vi "ULx Create Channel (DO-Digital Output).vi"(0 "task in":refnum<k24>, 5 "lines":refnum<k21>, 9 "line grouping":i32(ring)=1 items=["OneChannelForEachLine", "OneChannelForAllLines"], 11 "error in":errorcluster) -> (4 "task out":refnum<k24>, 15 "error out":errorcluster)   [LabVIEW 2020]
doc: "Creates channel(s) to generate digital signals. You can group digital lines into one digital channel or separate them into multiple digital channels. If you specify one or more entire ports in <B>lines</B> input by using port physical channel names, you cannot separate the ports into multiple channels. To separate ports into multiple channels, use this VI multiple times with a different port each time."
uses:
  C:/Users/William/Documents/LV 2020 builds/LeaktestDAQ/Source-v33/ULx_LV.dll
  ULx_LV.dll
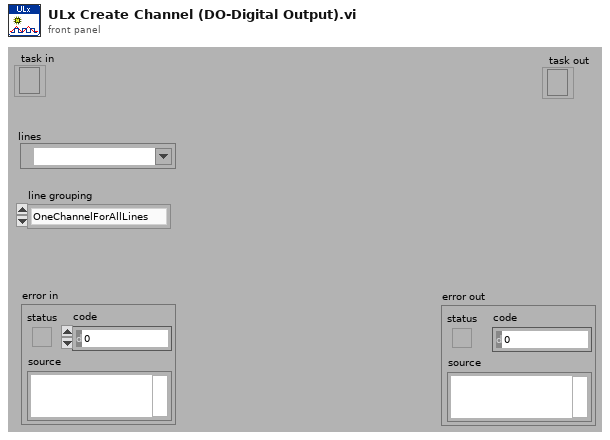
[diagram p1: front panel]
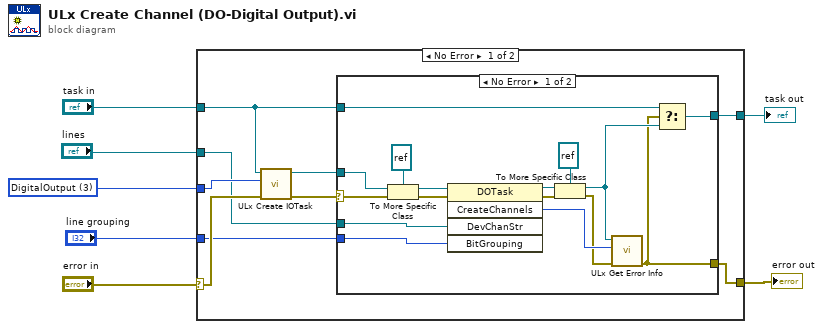
[diagram p0: block diagram]
diagram:
  w2 = 3 items=["AnalogInput", "AnalogOutput", "DigitalInput", "DigitalOutput", "CounterInput", "CounterOutput", "CompositeInput", "CompositeOutput", "TemperatureInput"] ("taskType")
  n1 = case shown="No Error" "error in" {
    selector: "error in" -> [w16 w36]
    tunnel: "task in" -> [w8 w35]
    tunnel: "lines" -> [w10 _]
    tunnel: w2 -> [w11 _]
    tunnel: [w14 w35] -> w5
    tunnel: [w13 w36] -> w4
    tunnel: "line grouping" -> [w9 _]
    frame No Error {
      n2 = call "ULx Create IOTask.vi"("error in"=w16, "taskType"=w11, "i/o task in"=w8) -> ("error out"=w15:errorcluster, "i/o task out"=w12:refnum<k24>)  [unwired: 7 in]
      n3 = case shown="No Error" w15 {
        selector: w15 -> [w30 w34]
        tunnel: [w17 w34] -> w13
        tunnel: [w20 w33] -> w14
        tunnel: w12 -> [w28 _]
        tunnel: w10 -> [w27 _]
        tunnel: w9 -> [w25 _]
        tunnel: w8 -> [w18 w33]
        frame No Error {
          n4 = To More Specific Class(target class=refnum<k24> refnum, reference=w28, error in=w30) -> (specific class reference=w31:refnum<k24>, error out=w29:errorcluster)
          n5 = invoke class="DOTask" method="CreateChannels"(reference=w31, error in=w29, "DevChanStr"=w27, "BitGrouping"=w25) -> (reference out=w23:refnum<k24>, error out=w22:errorcluster, "CreateChannels"=w26:i32)  [unwired: 1 in, 2 out]
          n6 = To More Specific Class(target class=refnum<k24> refnum, reference=w23, error in=w22) -> (specific class reference=w19:refnum<k24>, error out=w21:errorcluster)
          n7 = call "ULx Get Error Info.vi"("error in"=w21, "ErrorCode"=w26, "task in"=w19) -> ("error out"=w17:errorcluster)  [unwired: 8 in]
          n8 = Select(t=w18, s=w17, f=w19) -> (s? t:f=w20:refnum<k24>)
        }
        frame Error {
        }
      }
    }
    frame Error {
    }
  }
  "error out" <- w4
  "task out" <- w5
